vi "writeToXML.vi"(8 "error in (no error)":errorcluster, 10 "ClassLabel":string, 11 "GuideTargetClearOffset in":refnum<class "GuideTargetClearOffset.lvclass">) -> (0 "error out":errorcluster, 2 "XML out":string, 3 "GuideTargetClearOffset out":refnum<class "GuideTargetClearOffset.lvclass">)   [LabVIEW 2022 SP3, in "TCSDataDefinitions.lvlib" / "TCSCommand.lvlib" / "OffsetCommands.lvlib" / "GuideTargetClearOffset.lvclass"]
uses:
  GuideTargetClearOffset.lvclass
  ClearOffset/ClearOffset.lvclass
  <userlib>/Common/XML/XMLGenerator/XMLGenerator.lvclass
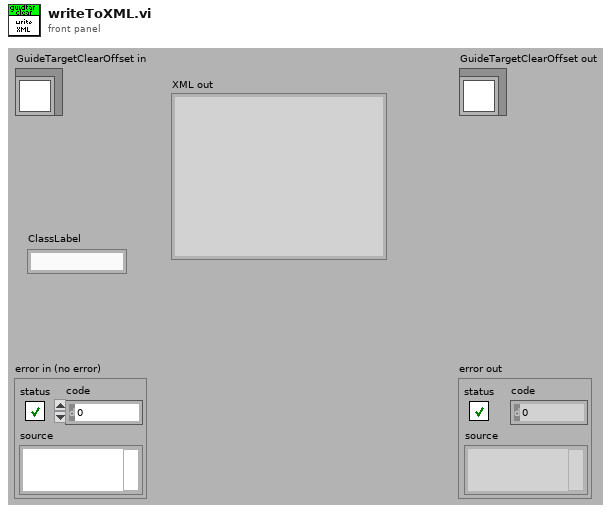
[diagram p1: front panel]
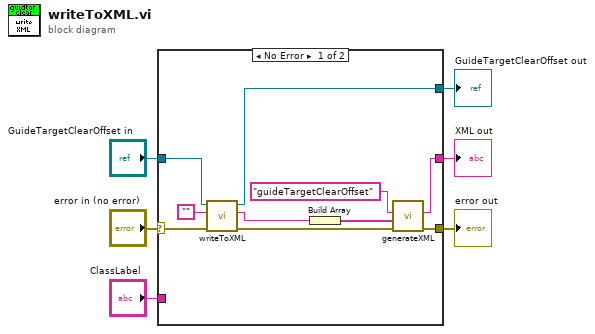
[diagram p0: block diagram]
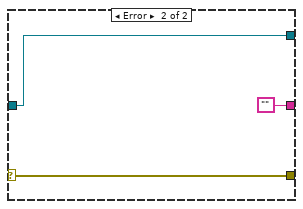
[diagram p2: hidden frame]
diagram:
  n1 = case shown="No Error" "error in (no error)" {
    selector: "error in (no error)" -> [w14 w19]
    tunnel: [w9 w19] -> w5
    tunnel: [w15 w18] -> w3
    tunnel: "GuideTargetClearOffset in" -> [w16 w18]
    tunnel: [w7 ""] -> w2
    tunnel: "ClassLabel" -> [_ _]
    frame No Error {
      n2 = call-parent "writeToXML.vi"("error in (no error)"=w14, "ClassLabel"="", "ClearOffset in"=w16) -> ("error out"=w10:errorcluster, "XML out"=w8:string, "ClearOffset out"=w15:refnum<class "GuideTargetClearOffset.lvclass">)  [unwired: 6 in]
      n3 = Build Array(w8) -> (w12:string[])
      n4 = call <userlib>:"generateXML.vi"("error in"=w10, "childrenXML"=w12, "elementName"="guideTargetClearOffset" ("ClassLabel")) -> ("error out"=w9:errorcluster, "XML out"=w7:string)  [unwired: 6 in, 1 out]
    }
    frame Error {
    }
  }
  "error out" <- w5
  "GuideTargetClearOffset out" <- w3
  "XML out" <- w2
